vi "Average5.vi"() -> ()   [LabVIEW 2016]
panel:
  in  "5":dbl
  out "average":dbl
  in  "4":dbl
  in  "3":dbl
  in  "2":dbl
  in  "1":dbl
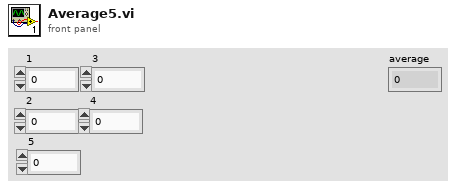
[diagram p1: front panel]
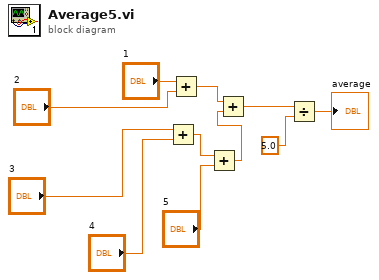
[diagram p0: block diagram]
diagram:
  n1 = Add(x="3", y="4") -> (x+y=w2:dbl)
  n2 = Add(x="1", y="2") -> (x+y=w11:dbl)
  n3 = Add(x=w2, y="5") -> (x+y=w3:dbl)
  n4 = Add(x=w11, y=w3) -> (x+y=w4:dbl)
  n5 = Divide(x=w4, y=5.0) -> (x/y=→"average":dbl)
